vi "Celsius2Far SubVI.vi"(1 "Celsius in":dbl) -> (0 "Fahrenheit Out":dbl)   [LabVIEW 2013]
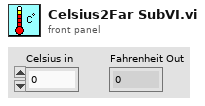
[diagram p1: front panel]
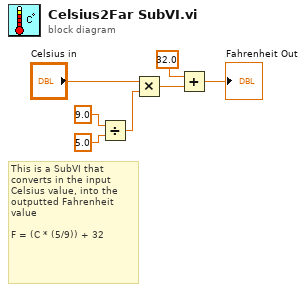
[diagram p0: block diagram]
diagram:
  # "This is a SubVI that converts in the input Celsius value, into the outputted Fahrenheit value\n\nF = (C * (5/9)) + 32"
  n1 = Divide(x=9.0, y=5.0) -> (x/y=w1:dbl)
  n2 = Multiply(x="Celsius in", y=w1) -> (x*y=w5:dbl)
  n3 = Add(x=32.0, y=w5) -> (x+y=→"Fahrenheit Out":dbl)
